vi "Subtract.vi"(10 "x":dbl, 11 "y":dbl) -> (2 "x-y":dbl)   [LabVIEW 2023]
panel:
  out "output cluster":cluster{"x":dbl, "y":dbl, dbl}
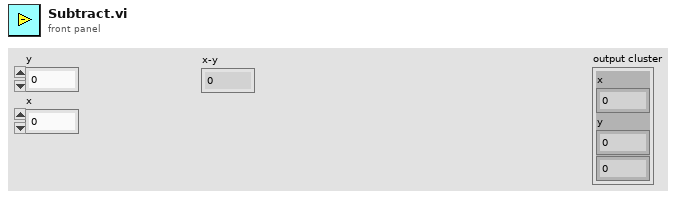
[diagram p1: front panel]
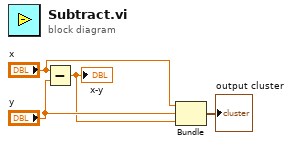
[diagram p0: block diagram]
diagram:
  n1 = Subtract(x="x", y="y") -> (x-y=w2:dbl)
  "x-y" <- w2
  n2 = Bundle("x"="x", "y"="y", w2) -> (→"output cluster":cluster{"x":dbl, "y":dbl, dbl})  [unwired: 1 in]
